vi "AIT 664 - Parse Channels.vi"(0 "Device Reference in":T8 format="%.0x", 1 "FIFO Index Queues":T13, 5 "End System Handle in":u64 format="%x", 11 "error in (no error)":errorcluster) -> (6 "Hardware Output - Tx Ports":T1[](array[typedef]) {"Message Settings"."Transmit Channel Data Reference" format="%.0x"; "Message Settings"."Queue Transmit Channel" format="%.0x"; "Message Settings"."Driver Data"."Num Bits" min=1 max=32; "Message Settings"."Block Data Refs"."Data Reference" format="%.0x"; "Rx Com Udp Port"."Handle" format="%08x"; "Tx Com Udp Port"."Handle" format="%08x"}, 8 "Hardware Input  -Rx Ports":T1[](array[typedef]) {"Message Settings"."Transmit Channel Data Reference" format="%.0x"; "Message Settings"."Queue Transmit Channel" format="%.0x"; "Message Settings"."Driver Data"."Num Bits" min=1 max=32; "Message Settings"."Block Data Refs"."Data Reference" format="%.0x"; "Rx Com Udp Port"."Handle" format="%08x"; "Tx Com Udp Port"."Handle" format="%08x"}, 15 "error out":errorcluster)   [LabVIEW 2013, in "AIT 664 Custom Device.lvlib"]
uses:
  AIT 664 Custom Device.lvlib
  <vilib>/NI Veristand/Custom Device API/Custom Device Item Ref.ctl
  RT Controls/FIFO Index Queues.ctl
  RT Controls/AIT 664 - RT Hardware Channel.ctl
  RT Controls/AIT 664 - RT Message Settings.ctl
  <vilib>/NI Veristand/Custom Device API/Block Data Reference.ctl
  <vilib>/NI Veristand/Custom Device API/Data Reference.ctl
  RT Controls/AIT 664 - Driver Data.ctl
  Controls and Global/Start Bit.ctl
  Controls and Global/Number of Bits.ctl
  <userlib>/ARINC 664/AIT 664 Controls/General/Message Port.ctl
  <userlib>/ARINC 664/AIT 664 Controls/General/Direction.ctl
  <userlib>/ARINC 664/AIT 664 Controls/General/Message Port Type.ctl
  System Explorer/Controls/664 - Sampling Type.ctl
  <vilib>/NI Veristand/Custom Device Tools/Custom Device Utility Library/NI VeriStand - Search for All Items by GUID.vi
  Controls and Global/Global.vi
  <vilib>/NI Veristand/Custom Device Tools/Custom Device Utility Library/Custom Device Utility Library.lvlib
  <vilib>/NI Veristand/Custom Device API/Custom Device API.lvlib
  <userlib>/ARINC 664/AIT 664 API.lvlib
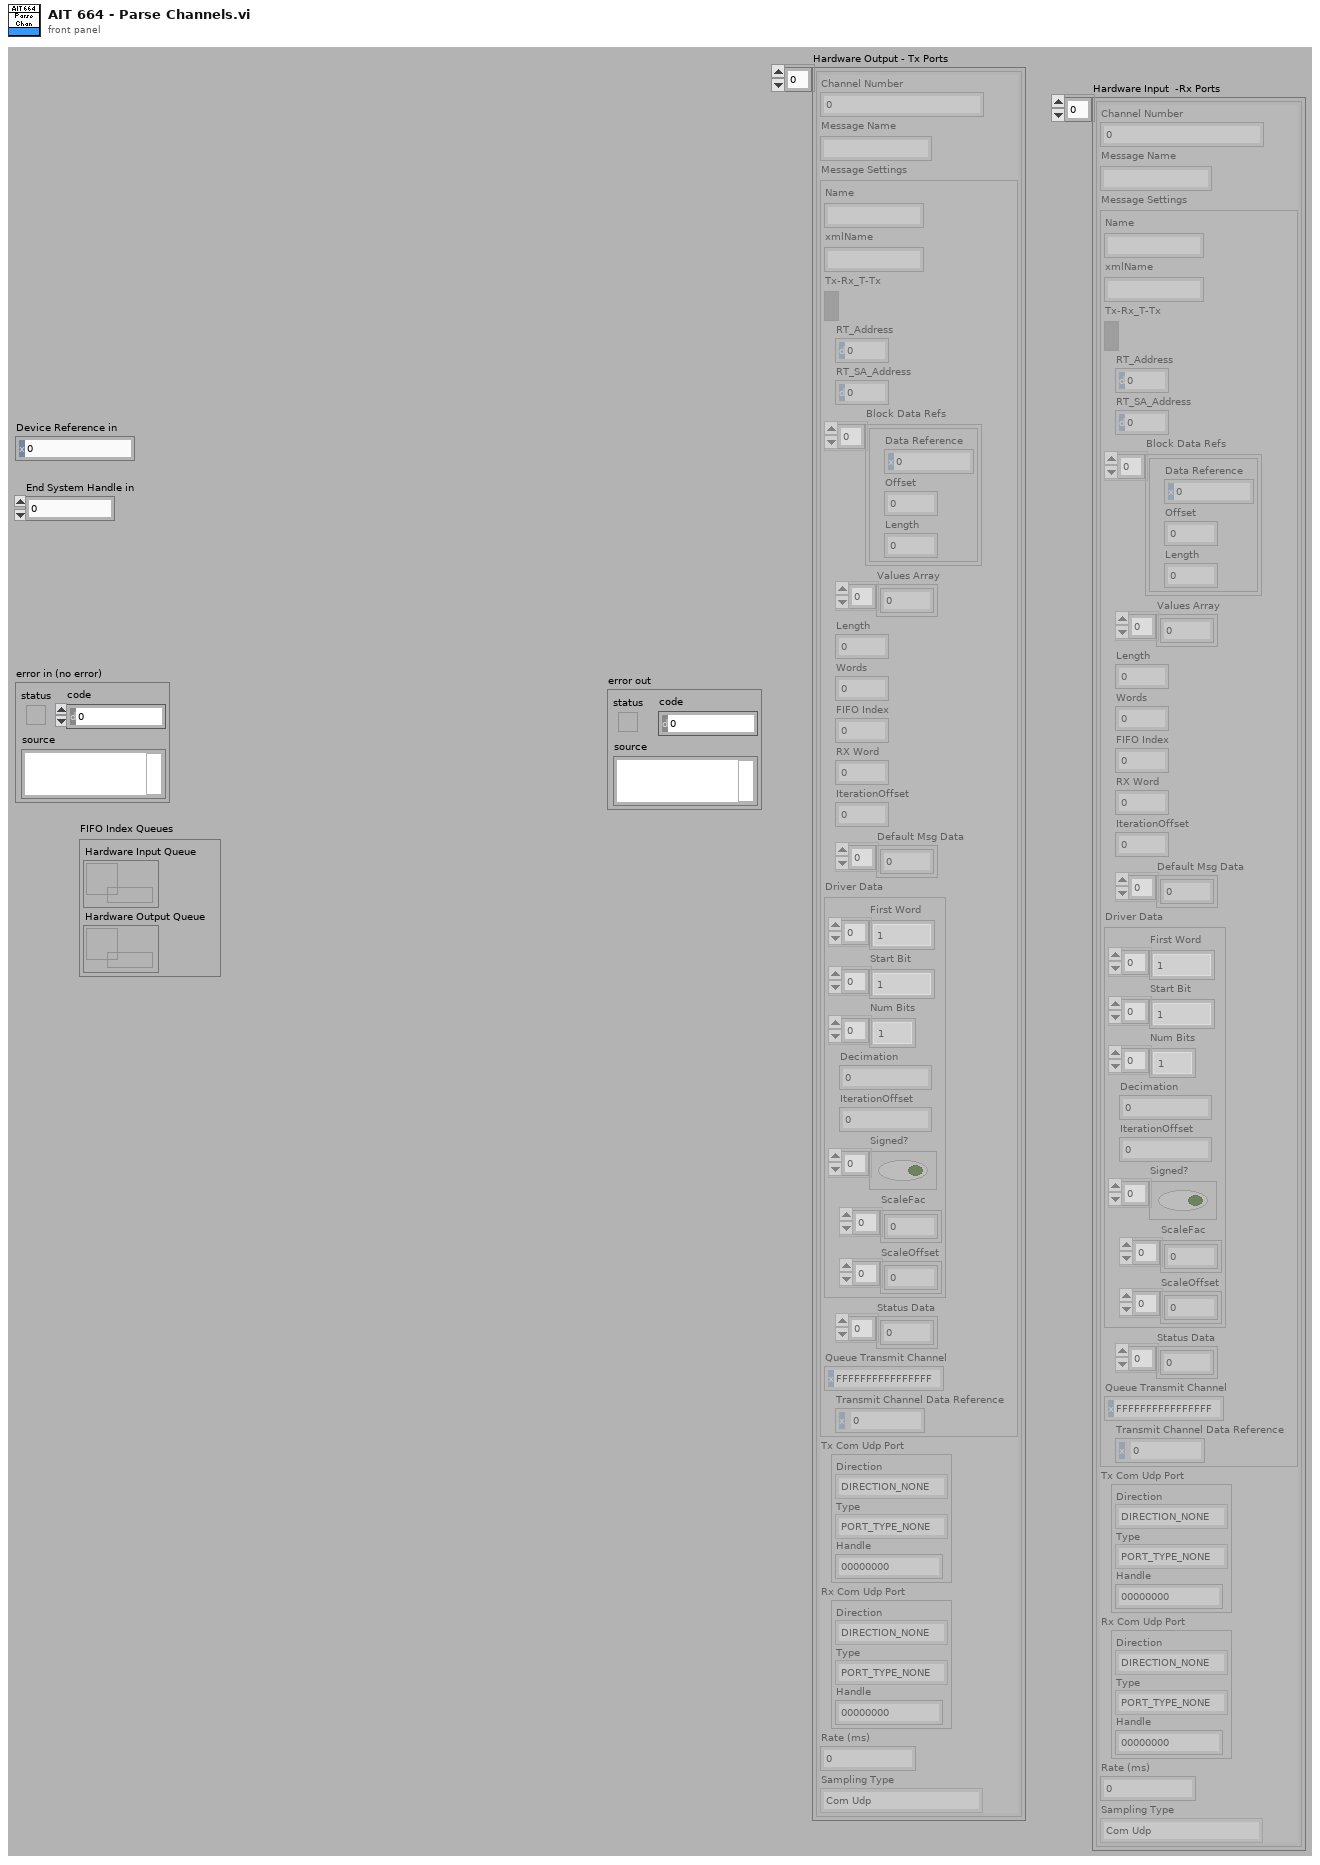
[diagram p1: front panel]
types:
  T1 = typedef "AIT 664 Custom Device.lvlib/AIT 664 - RT Hardware Channel.ctl" = cluster{"Channel Number":u16, "Message Name":string, "Message Settings":T2, "Tx Com Udp Port":T9, "Rx Com Udp Port":T9, "Rate (ms)":u32, "Sampling Type":T12}
  T2 = typedef "AIT 664 Custom Device.lvlib/AIT 664 - RT Message Settings.ctl" = cluster{"Name":string, "xmlName":string, "Tx-Rx_T-Tx":bool, "RT_Address":u8, "RT_SA_Address":u8, "Block Data Refs":T3[], "Values Array":dbl[], "Length":i32, "Words":i32, "FIFO Index":i32, "RX Word":u32, "IterationOffset":i32, "Default Msg Data":u8[], "Driver Data":T5, "Status Data":u32[], "Queue Transmit Channel":T8, "Transmit Channel Data Reference":T4}
  T3 = typedef "Custom Device API.lvlib/Block Data Reference.ctl" = cluster{"Data Reference":T4, "Offset":i32, "Length":i32}
  T4 = typedef "Custom Device API.lvlib/Data Reference.ctl" = i32
  T5 = typedef "AIT 664 Custom Device.lvlib/AIT 664 - Driver Data.ctl" = cluster{"First Word":T6[], "Start Bit":T6[], "Num Bits":T7[], "Decimation":i32, "IterationOffset":i32, "Signed?":bool[], "ScaleFac":dbl[], "ScaleOffset":dbl[]}
  T6 = typedef "AIT 664 Custom Device.lvlib/Start Bit.ctl" = i32
  T7 = typedef "AIT 664 Custom Device.lvlib/Number of Bits.ctl" = i32
  T8 = typedef "Custom Device API.lvlib/Custom Device Item Ref.ctl" = u64
  T9 = typedef "AIT 664 API.lvlib/Message Port.ctl" = cluster{"Direction":T10, "Type":T11, "Handle":u64}
  T10 = typedef "AIT 664 API.lvlib/Direction.ctl" = enum16{"DIRECTION_NONE", "DIRECTION_TX", "DIRECTION_RX"}
  T11 = typedef "AIT 664 API.lvlib/Message Port Type.ctl" = enum16{"PORT_TYPE_NONE", "COM_UDP", "SAP_UDP", "SAP_IP", "SAP_MAC", "COTS_MAC", "COTS_MAC_RAW"}
  T12 = typedef "AIT 664 Custom Device.lvlib/664 - Sampling Type.ctl" = enum16{"Com Udp", "Com Udp Queuing", "Sap Udp", "Sap Ip", "Sap Mac", "Unknown"}
  T13 = typedef "AIT 664 Custom Device.lvlib/FIFO Index Queues.ctl" = cluster{"Hardware Input Queue":refnum<queue>, "Hardware Output Queue":refnum<queue>}
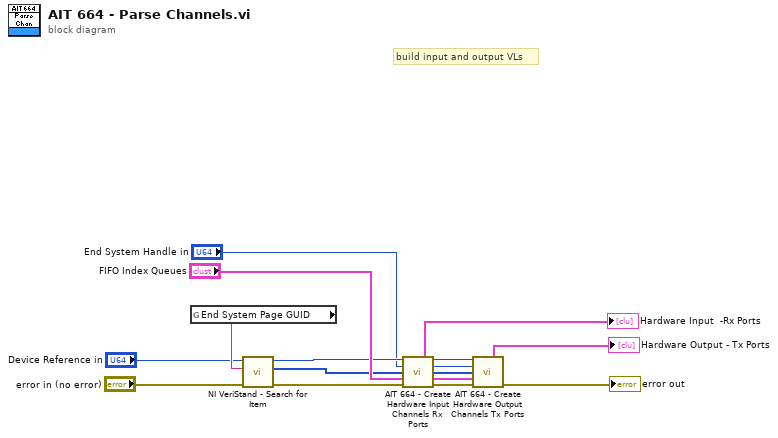
[diagram p0: block diagram]
diagram:
  # "build input and output VLs"
  n1 = global read "Global.vi" "End System Page GUID"() -> (w15:string)
  n2 = call-poly <vilib>:"NI VeriStand - Search for Item.vi"("error in"="error in (no error)", "Item GUID"=w15, "Section Ref in"="Device Reference in") -> ("error out"=w12:errorcluster, "Item Refs"=w8:T8[])  [unwired: 5 in, 2 out]
  n3 = call "AIT 664 - Create Hardware Input Channels Rx Ports.vi"("Device Reference in"="Device Reference in", "End System Handle in"="End System Handle in", "End System References in"=w8, "FIFO Index Queues in"="FIFO Index Queues", "error in (no error)"=w12) -> ("Hardware Input  -Rx Ports out"=→"Hardware Input  -Rx Ports":T1[], "Device Reference out"=w4:T8, "End System Handle out"=w3:u64, "End System References out"=w1:T8[], "FIFO Index Queues out"=w2:T13, "error out"=w11:errorcluster)  [unwired: 5 in]
  n4 = call "AIT 664 - Create Hardware Output Channels Tx Ports.vi"("Device Reference in"=w4, "End System Handle in"=w3, "End System References In"=w1, "FIFO Index Queues"=w2, "error in (no error)"=w11) -> ("Hardware Output - Tx Ports"=→"Hardware Output - Tx Ports":T1[], "error out"=→"error out":errorcluster)  [unwired: 9 in]
